vi "Remove_FF_lone_spikes.vi"(3 "ADC Frequency Hz":dbl=1000.0 format="%.2f", 4 "Bkgnd variance":dbl format="%.6f", 5 "AIC index":i32, 6 "Time Trace":dbl[](graph)) -> (0 "No Removed":i32, 2 "Filtered Time Trace":dbl[](graph))   [LabVIEW 2012]
uses:
  Globals/Meas_global.vi
  <vilib>/Analysis/NI_AALBase.lvlib
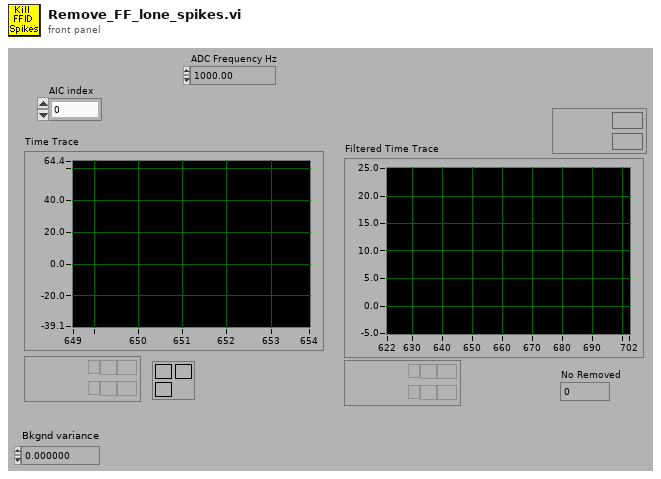
[diagram p1: front panel]
types:
  T1 = typedef "Analysis_info_cluster.ctl" = cluster{"Colour":u32, "Inst type":T2, "Inst name":string, "Symbol":string, "Code name":string, "Extra Info":string, "Inst Array":T3, "Extra Titles":string[], "Extra Values":string[], "U":dbl, "u^2":dbl, "u^3":dbl, "u^4":dbl, "Skew_u":dbl, "Kurt_u":dbl, "Sd Error in Mean":dbl, "% u'/U":dbl, "X":dbl, "Y":dbl, "Z":dbl, "Timescale integral to 25%":dbl, "Sd Error in Variance":dbl, "Calib File":path, "Calib Constants":dbl[], "Output Position":bool, "Full Stats":bool, "Av Sampling Rate":dbl, "Av No of Samples":dbl, "Total Meas Time (s)":dbl, "ADAM Ch Name":string}
  T2 = typedef "Inst_type.ctl" = enum16{"Propeller anemometer", "Raw voltage", "Pressure Transducer", "Pitot-static tube", "Preston tube", "Hot wire", "Cross wire 1", "Cross wire 2", "Generic Linear", "Generic Polynomial", "Generic BackPoly", "Fast FID", "Thermocouple", "Cold wire", "Pulsed Wire", "LDA Vel", "LDA Tran time", "LDA Arr time"}
  T3 = typedef "Instrument_Array.ctl" = enum16{"PWA", "LDA", "Analogue"}
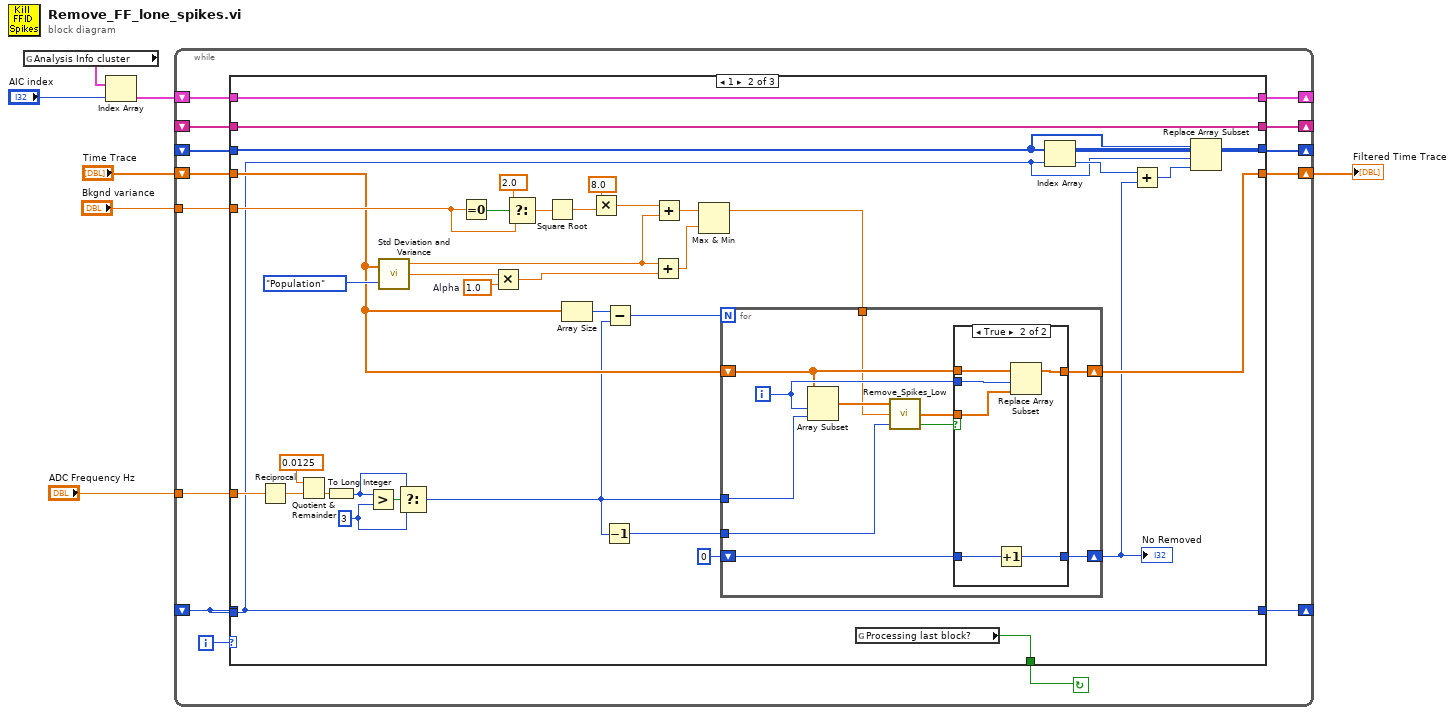
[diagram p0: block diagram]
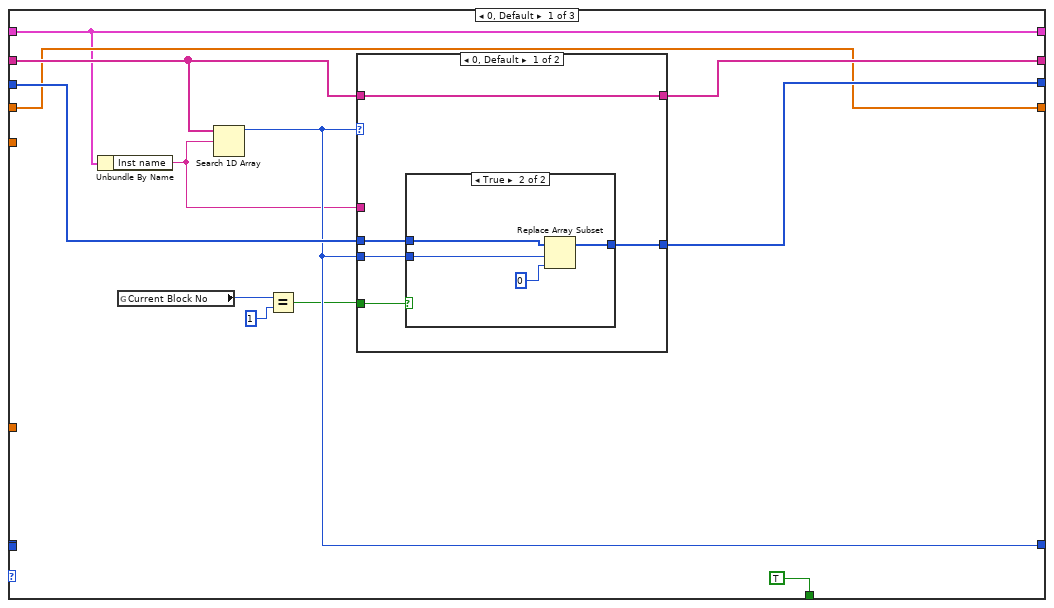
[diagram p2: hidden frame]
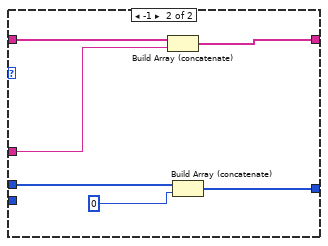
[diagram p4: hidden frame]
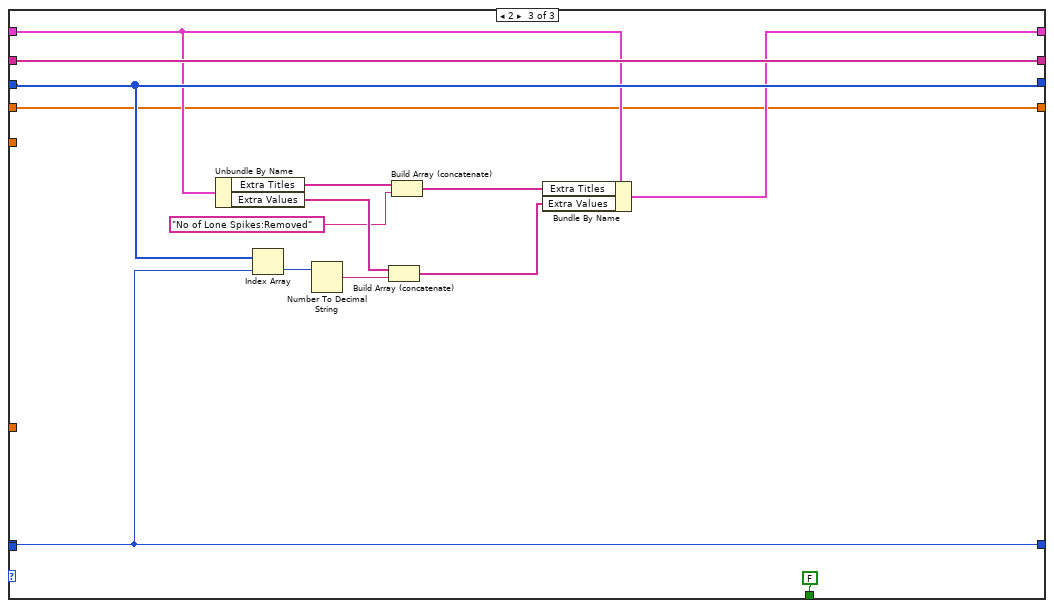
[diagram p6: hidden frame]
diagram:
  n1 = global read "Meas_global.vi" "Analysis Info cluster"() -> (w3:T1[])
  n2 = Index Array(array=w3, index="AIC index") -> (element=w1:T1)
  n3 = while {
    shift-left: _ -> [w18]
    shift-right: [w20] -> _
    shift-right: [w16] -> _
    shift-left: _ -> [w17]
    shift-right: [w14] -> _
    shift-left: _ -> [w15]
    shift-right: [w12] -> _
    shift-left: w1 -> [w13]
    tunnel: "Bkgnd variance" -> [w11]
    shift-right: [w9] -> w5
    shift-left: "Time Trace" -> [w10]
    tunnel: "ADC Frequency Hz" -> [w8]
    i -> [w21]
    stop <- w19 continue-if-true
    n4 = case shown="1" w21 {
      tunnel: [w26 w64 w118] -> w20
      tunnel: [TRUE w62 FALSE ("Processing last block?")] -> w19
      tunnel: w18 -> [_ _ w118]
      tunnel: w18 -> [_ w64 _]
      tunnel: w17 -> [w30 w80 w116]
      tunnel: [w29 w80 w116] -> w16
      tunnel: w15 -> [w28 w79 w115]
      tunnel: [w27 w77 w115] -> w14
      tunnel: w13 -> [w23 w76 w112]
      tunnel: [w23 w76 w114] -> w12
      tunnel: w11 -> [_ w75 _]
      tunnel: w10 -> [w24 w68 w107]
      tunnel: [w24 w63 w107] -> w9
      tunnel: w8 -> [_ w73 _]
      frame 0, Default {
        n5 = Unbundle By Name(w23) -> ("Inst name"=w22:string)
        n6 = global read "Meas_global.vi" "Current Block No"() -> (w32:i32)
        n7 = Search 1D Array(1D array=w30, element=w22) -> (index of element=w26:i32)  [unwired: 1 out]
        n8 = Equal?(x=w32, y=1) -> (x = y?=w25:bool)
        n9 = case shown="0, Default" w26 {
          tunnel: w30 -> [w38 w49]
          tunnel: w22 -> [_ w48]
          tunnel: [w38 w47] -> w29
          tunnel: w28 -> [w37 w46]
          tunnel: [w36 w45] -> w27
          tunnel: w26 -> [w35 _]
          tunnel: w25 -> [w34 _]
          frame 0, Default {
            n10 = case shown="True" w34 {
              tunnel: w37 -> [w39 w43]
              tunnel: [w39 w42] -> w36
              tunnel: w35 -> [_ w41]
              frame False {
              }
              frame True {
                n11 = Replace Array Subset(array=w43, new element=0, index=w41) -> (w42:i32[])
              }
            }
          }
          frame -1 {
            n12 = Build Array (concatenate)(w49, w48) -> (w47:string[])
            n13 = Build Array (concatenate)(w46, 0) -> (w45:i32[])
          }
        }
      }
      frame 1 {
        w58 = 3 ("y")
        w52 = 1.0  # Alpha
        n14 = Reciprocal(x=w73) -> (1/x=w71:dbl)
        n15 = Quotient & Remainder(x=0.0125, y=w71) -> (floor(x/y)=w70:dbl)  [unwired: 1 out]
        n16 = To Long Integer(number=w70) -> (32bit integer=w57:i32)
        n17 = Greater?(x=w57, y=w58) -> (0:w59:bool)
        n18 = call <vilib>:"Std Deviation and Variance.vi"("X"=w68, "Weighting (Sample)"=enum16{"Sample", "Population"}."Population") -> ("mean"=w54:dbl, "standard deviation"=w53:dbl)  [unwired: 1 out]
        n19 = Select(t=w57, s=w59, f=w58) -> (s? t:f=w56:i32)
        n20 = Equal To 0?(x=w75) -> (x = 0?=w86:bool)
        n21 = Multiply(x=w53, y=w52) -> (x*y=w55:dbl)
        n22 = Select(t=2.0, s=w86, f=w75) -> (s? t:f=w84:dbl)
        n23 = Square Root(x=w84) -> (sqrt(x)=w51:dbl)
        n24 = Array Size(array=w68) -> (size(s)=w67:i32)
        n25 = Multiply(x=8.0 ("y"), y=w51) -> (x*y=w87:dbl)
        n26 = Decrement(x=w56) -> (x-1=w69:i32)
        n27 = Subtract(x=w67, y=w56) -> (x-y=w66:i32)
        n28 = Add(x=w54, y=w55) -> (x+y=w81:dbl)
        n29 = Add(x=w87, y=w54) -> (x+y=w82:dbl)
        n30 = Max & Min(x=w82, y=w81) -> (max(x,y)=w65:dbl)  [unwired: 1 out]
        n31 = for {
          N: w66 -> [_]
          shift-right: [w91] -> w63
          shift-left: w68 -> [w92]
          tunnel: w56 -> [w98]
          tunnel: w69 -> [w97]
          tunnel: w65 -> [w90]
          shift-right: [w89] -> w61
          shift-left: 0 -> [w88]
          i -> [w94]
          n32 = Array Subset(array=w92, index=w94, length=w98) -> (w96:dbl[])
          n33 = call "Remove_Spikes_Low.vi"("index"=w97, "Background noise"=w90, "Time Trace"=w96) -> ("Spike"=w95:bool, "Filtered Time Trace"=w93:dbl[])  [unwired: 1 out]
          n34 = case shown="True" w95 {
            tunnel: w94 -> [_ w106]
            tunnel: w93 -> [_ w105]
            tunnel: w92 -> [w100 w104]
            tunnel: [w100 w103] -> w91
            tunnel: [w99 w101] -> w89
            tunnel: w88 -> [w99 w102]
            frame False {
            }
            frame True {
              n35 = Increment(x=w102) -> (x+1=w101:i32)
              n36 = Replace Array Subset(array=w104, new element=w105, index=w106) -> (w103:dbl[])
            }
          }
        }
        "No Removed" <- w61
        n37 = global read "Meas_global.vi" "Processing last block?"() -> (w62:bool)
        n38 = Index Array(array=w79, index=w64) -> (element=w78:i32)
        n39 = Add(x=w78, y=w61) -> (x+y=w74:i32)
        n40 = Replace Array Subset(array=w79, new element=w74, index=w64) -> (w77:i32[])
      }
      frame 2 {
        n41 = Unbundle By Name(w112) -> ("Extra Titles"=w111:string[], "Extra Values"=w110:string[])
        n42 = Index Array(array=w115, index=w118) -> (element=w117:i32)
        n43 = Number To Decimal String(number=w117) -> (decimal integer string=w119:string)  [unwired: 1 out]
        n44 = Build Array (concatenate)(w110, w119) -> (w109:string[])
        n45 = Build Array (concatenate)(w111, "No of Lone Spikes:Removed" ("format string")) -> (w113:string[])
        n46 = Bundle By Name(cluster=w112, "Extra Titles"=w113, "Extra Values"=w109) -> (w114:T1)
      }
    }
  }
  "Filtered Time Trace" <- w5
